vi "registerEvent.vi"(8 "error in (no error)":errorcluster, 10 "name":string, 11 "Event in":refnum<class "Event.lvclass">) -> (0 "error out":errorcluster, 3 "Event out":refnum<class "Event.lvclass">)   [LabVIEW 2009, in "Events.lvlib" / "Event.lvclass"]
uses:
  Event.lvclass
  Event.lvclass/Event.ctl
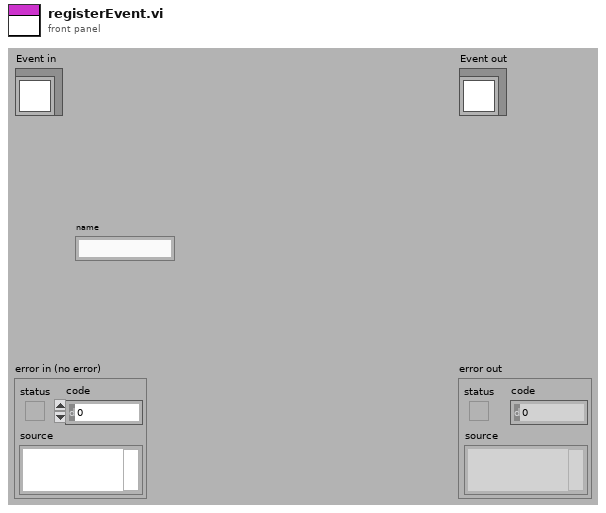
[diagram p1: front panel]
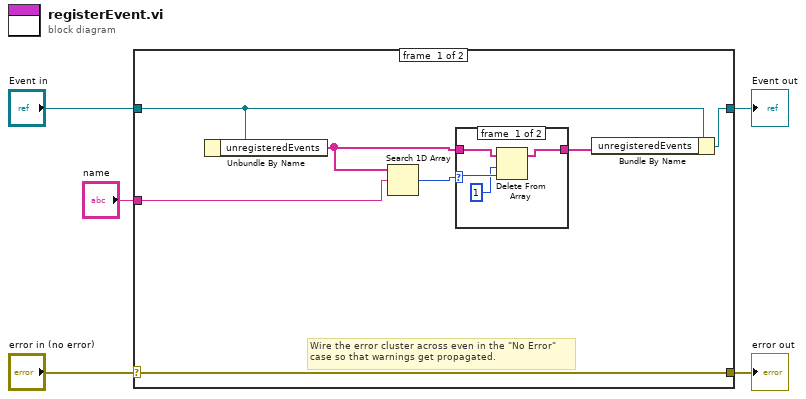
[diagram p0: block diagram]
diagram:
  n1 = case shown="No Error" "error in (no error)" {
    selector: "error in (no error)" -> [w12 w19]
    tunnel: [w12 w19] -> w4
    tunnel: [w6 w18] -> w2
    tunnel: "Event in" -> [w7 w18]
    tunnel: "name" -> [w11 _]
    frame #0 {
      # "Wire the error cluster across even in the \"No Error\"\ncase so that warnings get propagated."
      n2 = Unbundle By Name(w7) -> ("unregisteredEvents"=w9:string[])
      n3 = Search 1D Array(1D array=w9, element=w11) -> (index of element=w10:i32)  [unwired: 1 in]
      n4 = case shown="Default" w10 {
        selector: w10 -> [w15 _]
        tunnel: w9 -> [w16 w17]
        tunnel: [w13 w17] -> w8
        frame #0 {
          n5 = Delete From Array(array=w16, length=1, index=w15) -> (array with subset deleted=w13:string[])  [unwired: 1 out]
        }
        frame #1 {
        }
      }
      n6 = Bundle By Name(cluster=w7, "unregisteredEvents"=w8) -> (w6:refnum<class "Event.lvclass">)
    }
    frame #1 {
    }
  }
  "error out" <- w4
  "Event out" <- w2
